vi "gfitsio-get-image-type.vi"(8 "error in (no error)":errorcluster, 11 "gfits refnum":T1) -> (0 "error out":errorcluster, 2 "bitpix":T2 items=["<invalid type>"=0, "BYTE_IMG  (U8)"=8, "SHORT_IMG  (I16)"=16, "USHORT_IMG  (U16)"=20, "LONG_IMG  (I32)"=32, "ULONG_IMG  (U32)"=40, "FLOAT_IMG  (SGL)"=-32, "DOUBLE_IMG  (DBL)"=-64], 3 "dup gfits refnum":T1)   [LabVIEW 2011, in "gfitsio.lvlib"]
doc: "Get the equivalent data type of the image. If the image pixel values are scaled, with non-default values for the BZERO and BSCALE keywords, then the routine will return the 'equivalent' data type that is needed to store the scaled values. For example, if BITPIX = 16 and BSCALE = 0.1 then the equivalent data type is FLOAT_IMG. Similarly if BITPIX = 16, BSCALE = 1, and BZERO = 32768, then the the pixel values span the range of an unsigned short integer and the returned data type will be USHORT_IMG. Otherwise the physical data type of the FITS image, as given by the BITPIX keyword, is returned."
uses:
  gfitsio.lvlib
  cfitsio-bitpix.ctl
  gfitsio-refnum.ctl
  gfitsio.dll
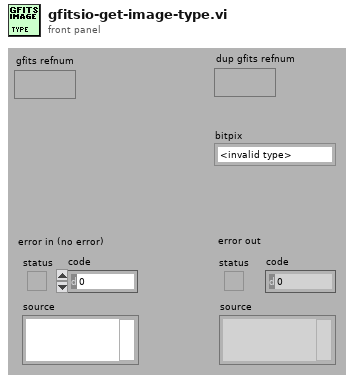
[diagram p1: front panel]
types:
  T1 = typedef "gfitsio.lvlib/gfitsio-refnum.ctl" = refnum<k1>
  T2 = typedef "gfitsio.lvlib/cfitsio-bitpix.ctl" = i32
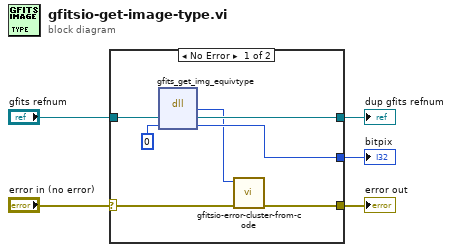
[diagram p0: block diagram]
diagram:
  n1 = case shown="No Error" "error in (no error)" {
    selector: "error in (no error)" -> [w7 w13]
    tunnel: "gfits refnum" -> [w12 w14]
    tunnel: [w11 _] -> w4
    tunnel: [w10 w14] -> w3
    tunnel: [w9 w13] -> w2
    frame No Error {
      n2 = dll-call lib="C:/BonOMM/BonOMM-SAOMM/SubVIs/gfitsio/gfitsio.dll" fn="gfits_get_img_equivtype"("gfits refnum"=w12, "bitpix"=0) -> (w8:i32, "gfits refnum"=w10:T1, "bitpix"=w11:i32)  [unwired: 3 in, 2 out]
      n3 = call "gfitsio-error-cluster-from-code.vi"("error in (no error)"=w7, "error code"=w8) -> ("error out"=w9:errorcluster)  [unwired: 9 in]
    }
    frame Error {
    }
  }
  "bitpix" <- w4
  "dup gfits refnum" <- w3
  "error out" <- w2
